vi "Create Sequence Parameter Assignment (Boolean Array).vi"(8 "error in (no error)":errorcluster, 10 "Value":bool[](array[boolean]), 11 "Parameter Name":string) -> (0 "error out":errorcluster, 3 "Sequence Parameter Assignment Ref":T1)   [LabVIEW 2020, in "NI_VS Sequence Execution Interface.lvlib"]
doc: "Assigns a value to a real-time sequence parameter. The value can be a constant value, data in a file, or a mapping to a channel in a system definition file. Use this VI to create parameter assignment references to use with the Create Sequence Call VI. \n\nWire data to the <B>Channel</B> input to determine the polymorphic instance to use or manually select the instance."
uses:
  <vilib>/NI VeriStand/Execution/SequenceExecutionInterface/NI_VS Sequence Execution Interface.lvlib
  <vilib>/NI VeriStand/Execution/SequenceExecutionInterface/Sequence Input Assignment Ref.ctl
  NationalInstruments.VeriStand.ClientAPI
  NationalInstruments.VeriStand.DataTypes
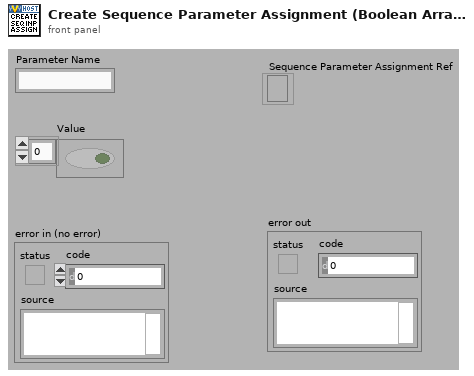
[diagram p1: front panel]
types:
  T1 = typedef "NI_VS Sequence Execution Interface.lvlib/Sequence Input Assignment Ref.ctl" = refnum<k24>
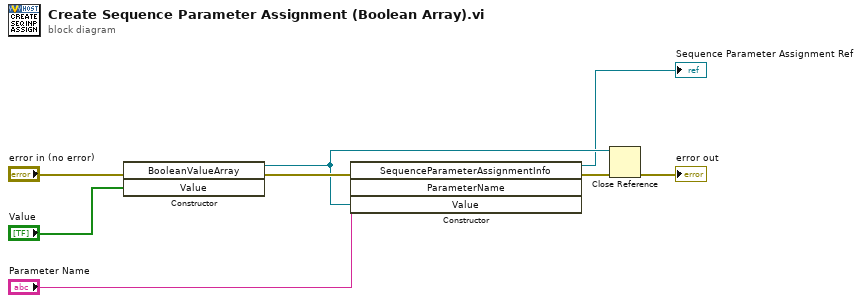
[diagram p0: block diagram]
diagram:
  n1 = constructor class="BooleanValueArray"(error in="error in (no error)", "Value"="Value") -> (reference out=w5:refnum<k24>, error out=w8:errorcluster)  [unwired: 2 in, 2 out]
  n2 = constructor class="SequenceParameterAssignmentInfo"(error in=w8, "ParameterName"="Parameter Name", "Value"=w5) -> (reference out=→"Sequence Parameter Assignment Ref":refnum<k24>, error out=w6:errorcluster)  [unwired: 2 in, 3 out]
  n3 = Close Reference(reference=w5, error in (no error)=w6) -> (error out=→"error out":errorcluster)
